vi "Audio Measurement with Filtering.vi"(5 "start":u32, 6 "units":T2={"SNR units"="dB", "THD+N units"="dB", "THD units"="dB", "Gain units"="dB"}, 7 "duration":u32, 8 "error in":errorcluster, 9 "filter settings":T3={"Highpass filter"="DC", "Lowpass filter"="No filter", "Weighting filter"="A-weighting"}, 10 "measurement settings":T4={"Band start"=20.0, "Band stop"=20000.0, "Amplitude"=1.0, "Frequency"=1000.0, "Full scale range"=3.16}, 11 "waveforms":waveform(dbl)[](array[waveform])) -> (0 "error out":errorcluster, 1 "spectra":cluster{"x0":dbl, "dx":dbl, "magnitude":dbl[]}[](array[cluster]), 2 "time domain":waveform(dbl)[](array[waveform]), 3 "results":T1(array[cluster]))   [LabVIEW 2021]
uses:
  controls/Single Tone Measurement Settings.ctl
  controls/Single Tone Filter Settings.ctl
  controls/Single Tone Units.ctl
  <vilib>/Waveform/WDTOps.llb/WDT Get Waveform Subset DBL.vi
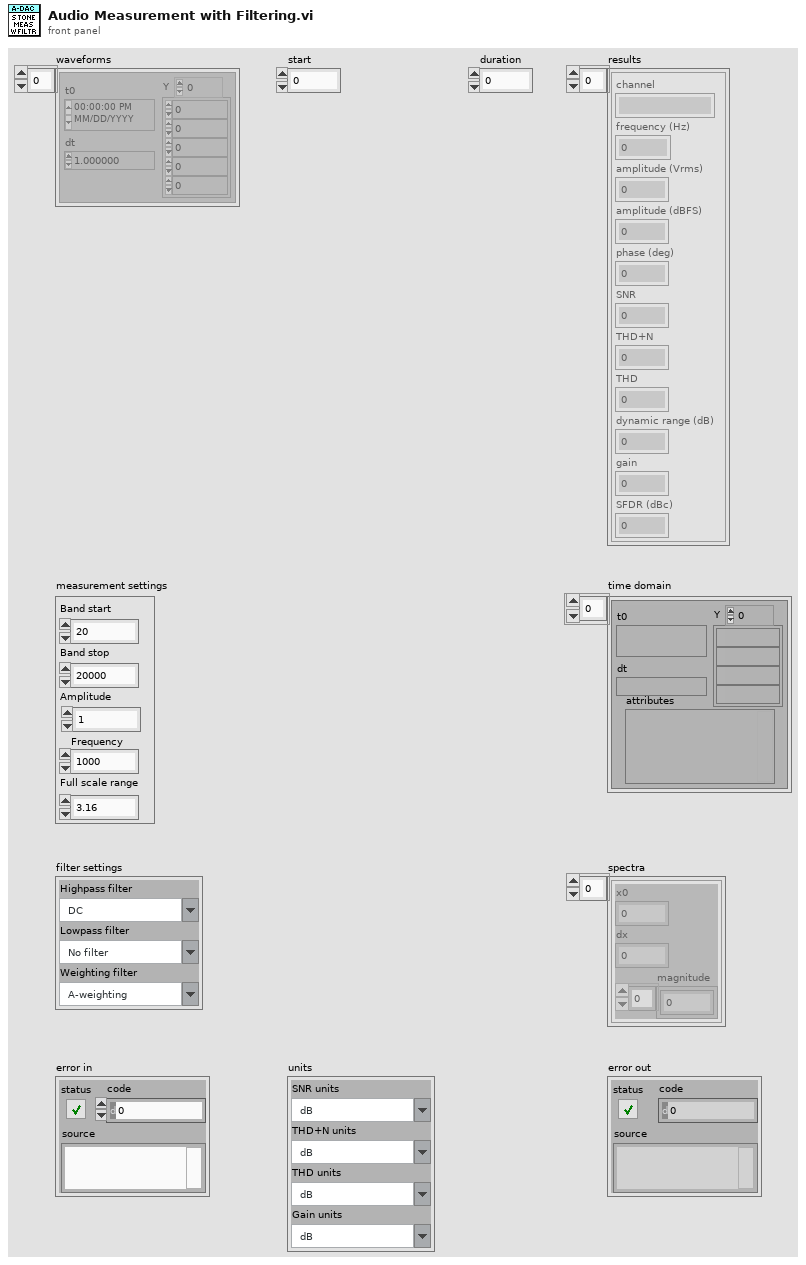
[diagram p1: front panel]
types:
  T1 = cluster{"channel":string, "frequency (Hz)":dbl, "amplitude (Vrms)":dbl, "amplitude (dBFS)":dbl, "phase (deg)":dbl, "SNR":dbl, "THD+N":dbl, "THD":dbl, "dynamic range (dB)":dbl, "gain":dbl, "SFDR (dBc)":dbl}[]
  T2 = typedef "Single Tone Units.ctl" = cluster{"SNR units":string, "THD+N units":string, "THD units":string, "Gain units":string}
  T3 = typedef "Single Tone Filter Settings.ctl" = cluster{"Highpass filter":string, "Lowpass filter":string, "Weighting filter":string}
  T4 = typedef "Single Tone Measurement Settings.ctl" = cluster{"Band start":dbl, "Band stop":dbl, "Amplitude":dbl, "Frequency":dbl, "Full scale range":dbl}
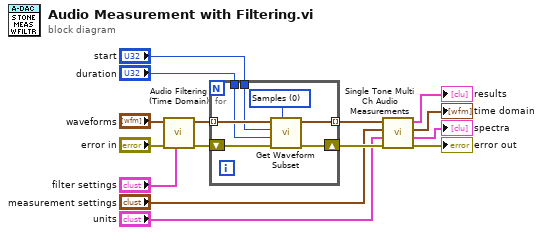
[diagram p0: block diagram]
diagram:
  n1 = call "Audio Filtering (Time Domain).vi"("Filter settings"="filter settings", "error in"="error in", "waveforms"="waveforms") -> ("error out"=w12:errorcluster, "time domain"=w13:waveform(dbl)[])  [unwired: 7 in]
  n2 = for {
    tunnel: w13 -> [w22] mode=indexing
    tunnel: [w21] -> w9 mode=indexing
    shift-right: [w18] -> w8
    shift-left: w12 -> [w19]
    tunnel: "start" -> [w17]
    tunnel: "duration" -> [w16]
    w20 = u16 0 items=["Samples", "Relative Time"] ("start/duration format")
    n3 = call-poly <vilib>:"Get Waveform Subset.vi"("start/duration format"=w20, "error in (no error)"=w19, "duration"=w16, "start samples/time"=w17, "waveform in"=w22) -> ("error out"=w18:errorcluster, "waveform out"=w21:waveform(dbl))  [unwired: 1 in, 2 out]
  }
  n4 = call "Single Tone Multi Ch Audio Measurements.vi"("error in"=w8, "units"="units", "measurement settings"="measurement settings", "waveforms"=w9) -> ("error out"=→"error out":errorcluster, "spectra"=→"spectra":cluster{"x0":dbl, "dx":dbl, "magnitude":dbl[]}[], "waveforms"=→"time domain":waveform(dbl)[], "results"=→"results":T1)  [unwired: 4 in]
